vi "FindRealObject.vi"(0 "flattened remote ref":string, 5 "error in (no error)":errorcluster) -> (12 "G#DebugServer ref":refnum<class "G#Object.lvclass">, 14 "real object ref":refnum<class "G#Object.lvclass">, 15 "not found":bool, 16 "in client memory?":bool, 19 "error out":errorcluster)   [LabVIEW 2017, in "G#DebugServer.lvclass"]
doc: "Finds the real object."
uses:
  <vilib>/addons/_AddQ/G#DebugServer/G#DebugServer.lvclass
  <vilib>/addons/_AddQ/G#Object/G#Object.lvclass
  C:/Program Files (x86)/National Instruments/LabVIEW 2017/vi.lib/addons/_AddQ/G#Object/G#Object.lvclass
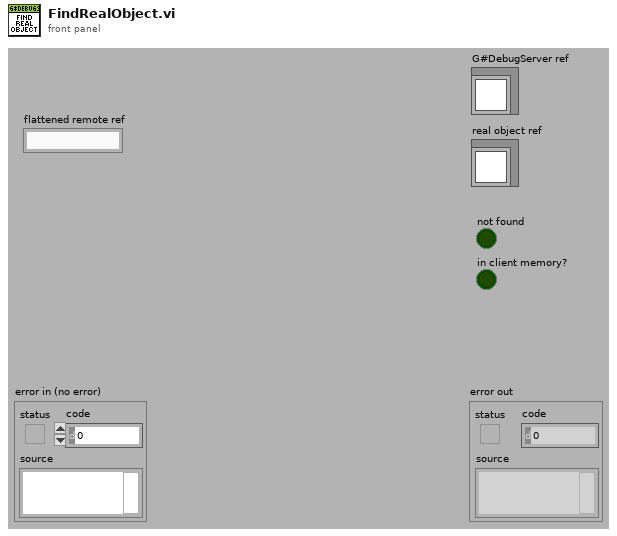
[diagram p1: front panel]
types:
  T1 = cluster{bool, "G#Object reference in":refnum<class "G#Object.lvclass">}
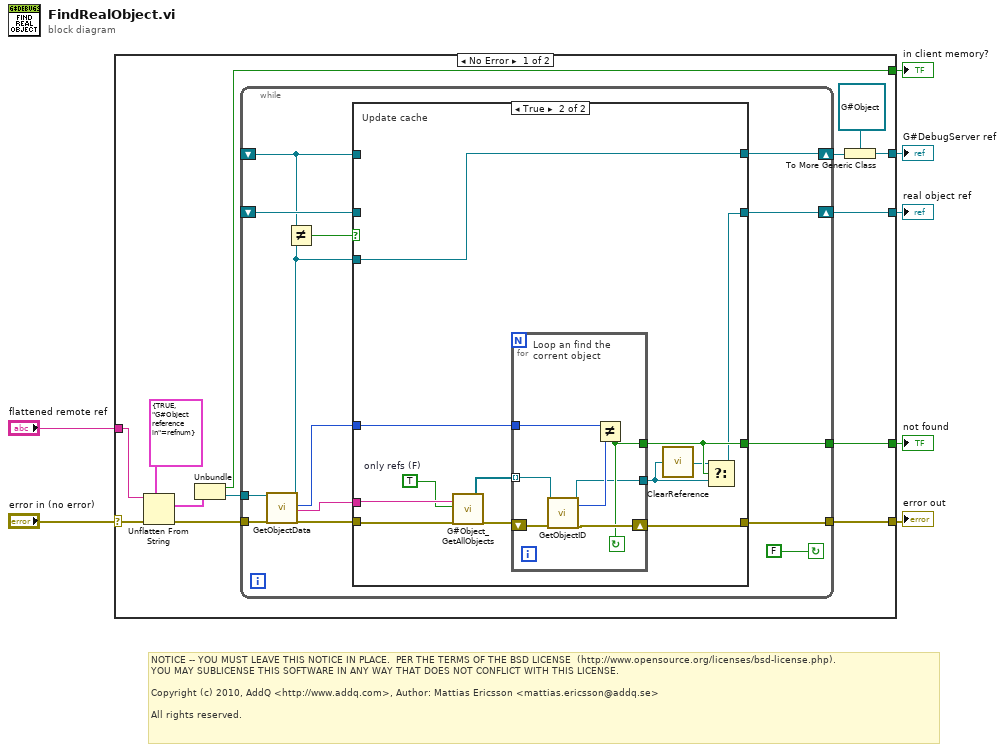
[diagram p0: block diagram]
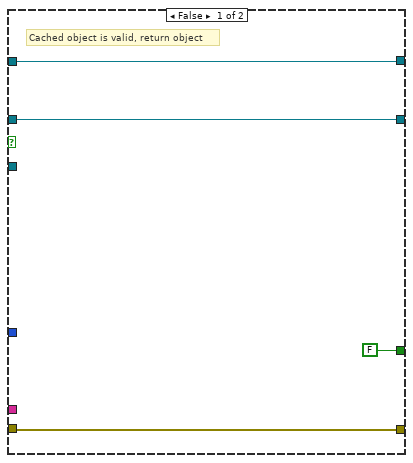
[diagram p2: hidden frame]
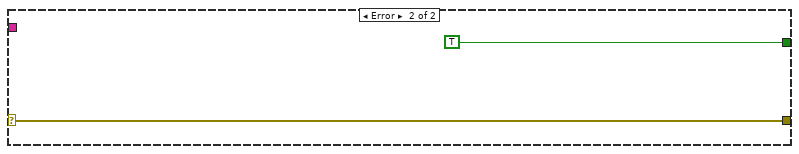
[diagram p3: hidden frame]
diagram:
  # "NOTICE -- YOU MUST LEAVE THIS NOTICE IN PLACE.  PER THE TERMS OF THE BSD LICENSE  (http://www.opensource.org/licenses/bsd-license.php).\nYOU MAY SUBLICENSE THIS SOFTWARE IN ANY WAY THAT DOES NOT CONFLICT WITH THIS LICENSE.\n\nCopyright (c) 2010, AddQ <http://www.addq.com>, Author: Mattias Ericsson <mattias.ericsson@addq.se>\n\nAll rights reserved."
  n1 = case shown="No Error" "error in (no error)" {
    selector: "error in (no error)" -> [w17 w59]
    tunnel: [w20 w59] -> w6
    tunnel: [w19 TRUE] -> w5
    tunnel: [w18 _] -> w4
    tunnel: "flattened remote ref" -> [w15 _]
    tunnel: [w12 _] -> w2
    tunnel: [w8 _] -> w1
    frame No Error {
      n2 = Unflatten From String(type=T1 {TRUE, "G#Object reference in"=refnum}, binary string=w15, error in (no error)=w17) -> (value=w10:T1, error out=w16:errorcluster)  [unwired: 2 in, 1 out]
      n3 = Unbundle(w10) -> (w8:bool, "G#Object reference in"=w9:refnum<class "G#Object.lvclass">)
      n4 = while {
        tunnel: w16 -> [w34]
        tunnel: [w25] -> w20
        shift-right: [w31] -> w14
        shift-left: _ -> [w22]
        shift-right: [w23] -> w18
        shift-left: _ -> [w26]
        tunnel: [w24] -> w19
        tunnel: w9 -> [w21]
        stop <- FALSE continue-if-true
        n5 = call <vilib>:"GetObjectData.vi"("remote ref"=w21, "error in (no error)"=w34) -> ("G#DebugServer reference out"=w33:refnum<class "G#DebugServer.lvclass">, "ObjectID"=w29:u32, "FullClassName"=w28:string, "error out"=w27:errorcluster)  [unwired: 13 in, 1 out]
        n6 = Not Equal?(x=w22, y=w33) -> (x != y?=w32:bool)
        n7 = case shown="True" w32 {
          tunnel: w33 -> [_ w50]
          tunnel: [w38 w50] -> w31
          tunnel: w22 -> [w38 _]
          tunnel: w29 -> [_ w44]
          tunnel: w28 -> [_ w48]
          tunnel: w27 -> [w36 w49]
          tunnel: w26 -> [w37 _]
          tunnel: [w36 w43] -> w25
          tunnel: [FALSE w42] -> w24
          tunnel: [w37 w39] -> w23
          frame False {
            # "Cached object is valid, return object"
          }
          frame True {
            w47 = TRUE  # only refs (F)
            # "Update cache"
            n8 = call <vilib>:"G#Object_GetAllObjects.vi"("full class name (\"\")"=w48, "only refs (F)"=w47, "error in (no error)"=w49) -> ("all refs"=w46:refnum<class "G#Object.lvclass">[], "error out"=w45:errorcluster)  [unwired: 13 in, 2 out]
            n9 = for {
              tunnel: w46 -> [w56] mode=indexing
              shift-right: [w53] -> w43
              shift-left: w45 -> [w57]
              tunnel: w44 -> [w55]
              tunnel: [w52] -> w42
              tunnel: [w51] -> w40
              stop <- w52 continue-if-true
              # "Loop an find the\ncorrent object"
              n10 = call-dynamic "GetObjectID.vi"("reference in"=w56, "error in (no error)"=w57) -> ("reference out"=w51:refnum<class "G#Object.lvclass">, "object ID"=w54:u32, "error out"=w53:errorcluster)  [unwired: 15 in]
              n11 = Not Equal?(x=w55, y=w54) -> (x != y?=w52:bool)
            }
            n12 = call-dynamic "ClearReference.vi"("reference in"=w40) -> ("reference out"=w41:refnum<class "G#Object.lvclass">)
            n13 = Select(t=w41, s=w42, f=w40) -> (s? t:f=w39:refnum<class "G#Object.lvclass">)
          }
        }
      }
      n14 = To More Generic Class(target class=refnum<class "G#Object.lvclass"> refnum ("G#Object reference in"), reference=w14) -> (generic class reference=w12:refnum<class "G#Object.lvclass">)
    }
    frame Error {
    }
  }
  "error out" <- w6
  "not found" <- w5
  "real object ref" <- w4
  "G#DebugServer ref" <- w2
  "in client memory?" <- w1
